vi "xy Exp. Data_in V1.00.vi"(0 "X-axis row":dbl[](array[numeric]) format="%.2f", 1 "Data row":dbl[](array[numeric]) format="%.2f", 3 "Continue?":bool=TRUE) -> (5 "X-Axis Array":dbl[][](array[numeric]) format="%.2f", 6 "Data Array":dbl[][](array[numeric]) format="%.2f")   [LabVIEW 2020]
uses:
  Globals and TypeDefs/Global Varibal Control.vi
  ExperimentLogGlobal.vi
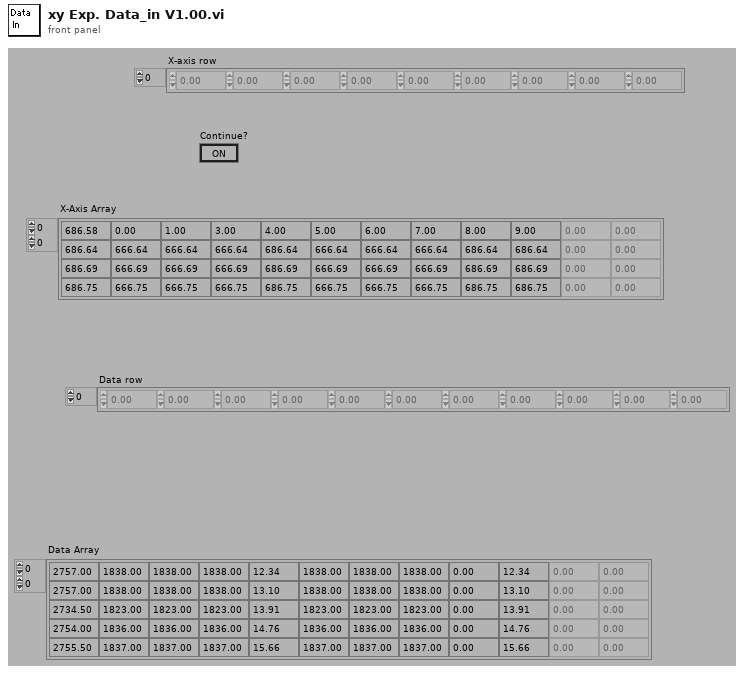
[diagram p1: front panel]
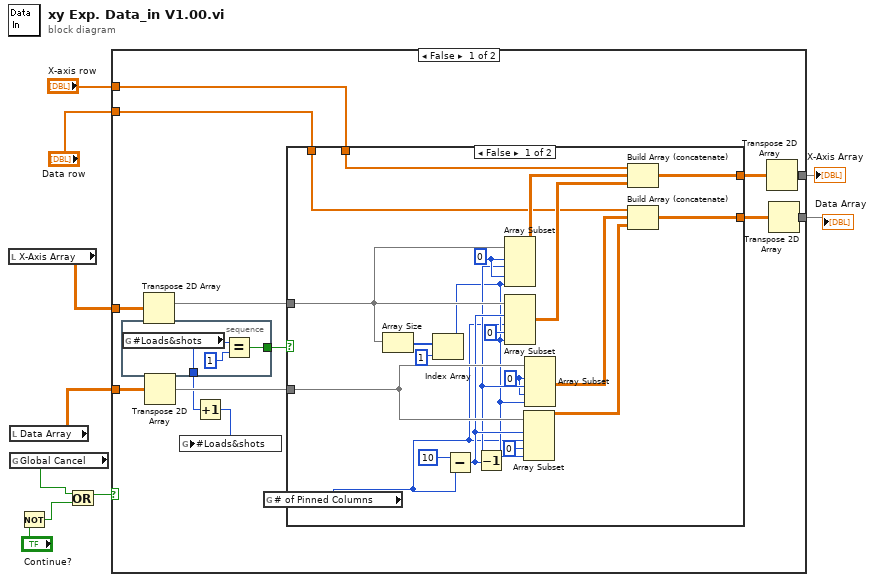
[diagram p0: block diagram]
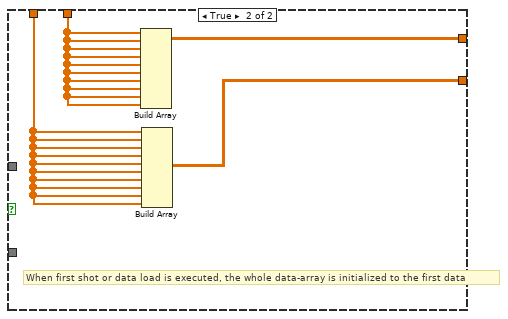
[diagram p2: hidden frame]
diagram:
  n1 = local read "X-Axis Array"() -> (w6:dbl[][])
  n2 = local read "Data Array"() -> (w2:dbl[][])
  n3 = global read "Global Varibal Control.vi" "Global Cancel"() -> (w1:bool)
  n4 = Not(x="Continue?") -> (.not. x?=w4:bool)
  n5 = Or(x=w1, y=w4) -> (x .or. y?=w3:bool)
  n6 = case shown="False" w3 {
    tunnel: [w21 w53] -> w10
    tunnel: [w20 w52] -> w9
    tunnel: "X-axis row" -> [w17 _]
    tunnel: "Data row" -> [w16 _]
    tunnel: w6 -> [w15 w53]
    tunnel: w2 -> [w14 w52]
    frame False {
      n7 = stacked-sequence {
        tunnel: [w24] -> w13
        tunnel: [w26] -> w12
        frame #0 {
          n8 = global read "ExperimentLogGlobal.vi" "#Loads&shots"() -> (w26:u32)
          n9 = Equal?(x=w26, y=u32 1) -> (x = y?=w24:bool)
        }
      }
      n10 = Transpose 2D Array(2D array=w15) -> (transposed array=w19:dbl[][])
      n11 = Transpose 2D Array(2D array=w14) -> (transposed array=w18:dbl[][])
      n12 = Increment(x=w12) -> (x+1=w11:u32)
      n13 = global write "ExperimentLogGlobal.vi" "#Loads&shots"(w11) -> ()
      n14 = case shown="False" w13 {
        tunnel: [w47 w49] -> w23
        tunnel: [w46 w48] -> w22
        tunnel: w19 -> [w40 _]
        tunnel: w18 -> [w38 _]
        tunnel: w17 -> [w29 w51]
        tunnel: w16 -> [w28 w50]
        frame False {
          w32 = 0
          w35 = 0
          n15 = global read "Global Varibal Control.vi" "# of Pinned Columns"() -> (w27:u8)
          n16 = Array Size(array=w40) -> (size(s)=w44:i32[])
          n17 = Index Array(array=w44, index=1) -> (element=w31:i32)
          n18 = Subtract(x=10, y=w27) -> (x-y=w36:i32)
          n19 = Decrement(x=w36) -> (x-1=w33:i32)
          n20 = Array Subset(array=w40, index (row)=w35, length (row)=w33, index (col)=w35, length (col)=w31) -> (w43:dbl[][])
          n21 = Array Subset(array=w40, index (row)=w36, length (row)=w27, index (col)=0, length (col)=w31) -> (w39:dbl[][])
          n22 = Array Subset(array=w38, index (row)=w36, length (row)=w27, index (col)=0, length (col)=w31) -> (w37:dbl[][])
          n23 = Array Subset(array=w38, index (row)=w32, length (row)=w33, index (col)=w32, length (col)=w31) -> (w42:dbl[][])
          n24 = Build Array (concatenate)(w29, w43, w39) -> (w47:dbl[][])
          n25 = Build Array (concatenate)(w28, w42, w37) -> (w46:dbl[][])
        }
        frame True {
          # "When first shot or data load is executed, the whole data-array is initialized to the first data"
          n26 = Build Array(w51, w51, w51, w51, w51, w51, w51, w51, w51, w51) -> (w49:dbl[][])
          n27 = Build Array(w50, w50, w50, w50, w50, w50, w50, w50, w50, w50) -> (w48:dbl[][])
        }
      }
      n28 = Transpose 2D Array(2D array=w23) -> (transposed array=w21:dbl[][])
      n29 = Transpose 2D Array(2D array=w22) -> (transposed array=w20:dbl[][])
    }
    frame True {
    }
  }
  "Data Array" <- w9
  "X-Axis Array" <- w10
